vi "Create Session.vi"(5 "Session in":refnum<class "Session.lvclass">, 8 "error in (no error)":errorcluster, 9 "Request":refnum<queue>, 11 "Connection":refnum<class "Connection.lvclass">) -> (0 "error out":errorcluster, 3 "Session":refnum<class "Session.lvclass">)   [LabVIEW 2013, in "MQTT Base.lvlib" / "Session.lvclass"]
uses:
  Session.lvclass
  <vilib>/LabVIEW Open Source Project/Connection/Connection/Connection.lvclass
  Base Class/Request -- cluster.ctl
  <vilib>/LabVIEW Open Source Project/MQTT Control Packets/Control Packets/ControlPacket/ControlPacket.lvclass
  Base Class/Response -- cluster.ctl
  Session State -- cluster.ctl
  <vilib>/LabVIEW Open Source Project/MQTT Control Packets/Control Packets/SUBSCRIBE/Topic Subscription -- cluster.ctl
  <vilib>/LabVIEW Open Source Project/MQTT Control Packets/Control Packets/ControlPacket/QualityOfService -- enum.ctl
  <vilib>/LabVIEW Open Source Project/MQTT Control Packets/Control Packets/ControlPacket/Pending Transmission -- cluster.ctl
  Session.lvclass/Session.ctl
  Base Class/MQTT_Base.lvclass
  <vilib>/LabVIEW Open Source Project/MQTT Control Packets/Control Packets/SUBSCRIBE/SUBSCRIBE.lvclass
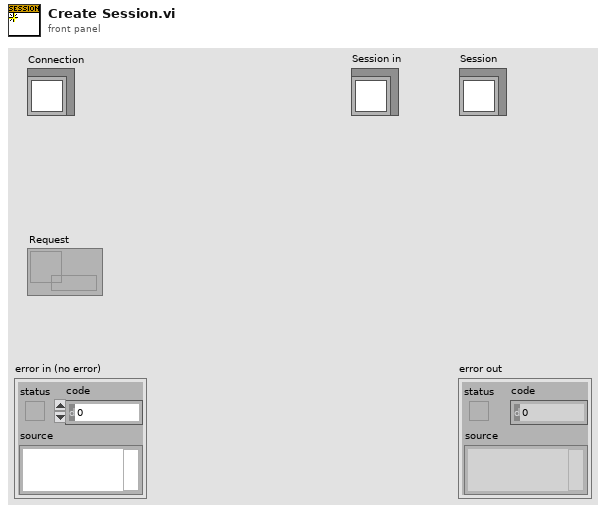
[diagram p1: front panel]
types:
  T1 = typedef "MQTT Base.lvlib/MQTT_Base.lvclass/Response -- cluster.ctl" = cluster{"Packet":refnum<class "ControlPacket.lvclass">, "Protocol Error":errorcluster, "disconnect session":bool, "[ACK]":refnum<notifier>[]}
  T2 = typedef "MQTT Base.lvlib/Session.lvclass/Session State -- cluster.ctl" = cluster{"CleanSession":bool, "Client ID":string, "Subscriptions":T3[], "Pending Transmissions":T5[], "Pending ACK map":variant}
  T3 = typedef "MQTT_Control_Packets.lvlib/SUBSCRIBE.lvclass/Topic Subscription -- cluster.ctl" = cluster{"Topic Filter":string, "QoS":T4}
  T4 = typedef "MQTT_Control_Packets.lvlib/ControlPacket.lvclass/QualityOfService -- enum.ctl" = enum16{"0 (At Most Once)", "1 (At Least Once)", "2 (Exactly Once)"}
  T5 = typedef "MQTT_Control_Packets.lvlib/ControlPacket.lvclass/Pending Transmission -- cluster.ctl" = cluster{"Message":refnum<class "ControlPacket.lvclass">, "QoS":T4, "Tx-Rx":bool}
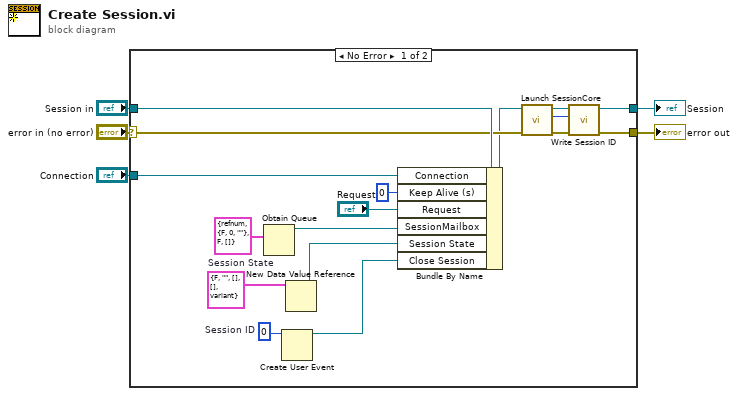
[diagram p0: block diagram]
diagram:
  n1 = case shown="No Error" "error in (no error)" {
    selector: "error in (no error)" -> [w16 w23]
    tunnel: [w10 w23] -> w4
    tunnel: [w15 w22] -> w2
    tunnel: "Session in" -> [w20 w22]
    tunnel: "Connection" -> [w18 _]
    frame No Error {
      w8 = 0  # Session ID
      w14 = T2 {"CleanSession"=FALSE, "Client ID"="", "Subscriptions"=[], "Pending Transmissions"=[], "Pending ACK map"=variant}  # Session State
      n2 = Obtain Queue(element data type=T1 {"Packet"=refnum, "Protocol Error"={"status"=FALSE, "code"=0, "source"=""}, "disconnect session"=FALSE, "[ACK]"=[]} ("Response")) -> (queue out=w21:refnum<queue>)  [unwired: 4 in, 2 out]
      n3 = Create User Event(user event datatype=w8) -> (user event=w7:refnum<user-event>)  [unwired: 1 in, 1 out]
      n4 = New Data Value Reference(data value=w14) -> (data value reference=w13:refnum<data-value>)  [unwired: 1 in, 1 out]
      n5 = Bundle By Name(cluster=w20, "Connection"=w18, "Keep Alive (s)"=0, "Request"="Request", "SessionMailbox"=w21, "Session State"=w13, "Close Session"=w7) -> (w9:refnum<class "Session.lvclass">)
      n6 = call "Launch SessionCore.vi"("error in (no error)"=w16, "Session in"=w9) -> ("error out"=w10:errorcluster, "Session ID"=w12:i32, "Session out"=w11:refnum<class "Session.lvclass">)  [unwired: 7 in]
      n7 = call "Write Session ID.vi"("Session ID"=w12, "Session in"=w11) -> ("Session out"=w15:refnum<class "Session.lvclass">)  [unwired: 8 in, 1 out]
    }
    frame Error {
    }
  }
  "error out" <- w4
  "Session" <- w2
